vi "UI Enable & Disable.vi"(7 "Mode":T2(ring), 8 "error in (no error)":errorcluster, 11 "Ctl Refs In":T1) -> (0 "error out":errorcluster, 3 "Ctl Refs Out":T1)   [LabVIEW 2015]
doc: "VI that manages enabling & disabling certain portions of the UI under different sets of conditions."
uses:
  Type Defs/Control Refs.ctl
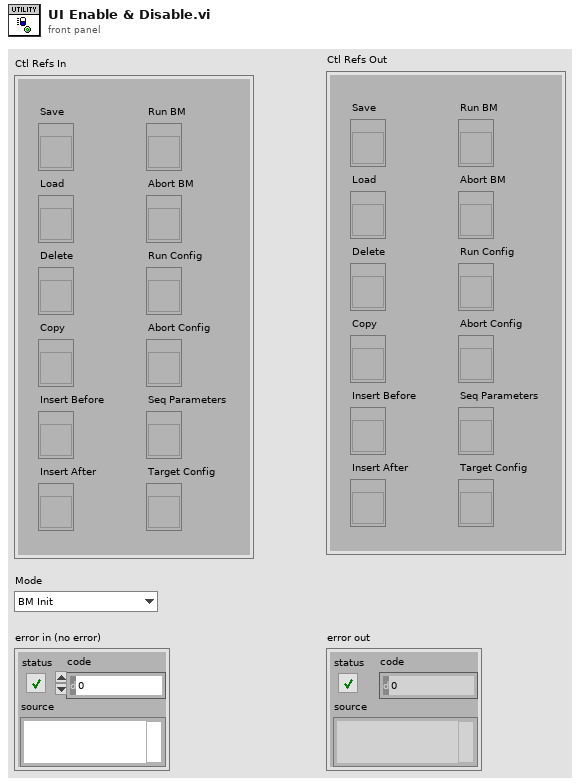
[diagram p1: front panel]
types:
  T1 = typedef "Control Refs.ctl" = cluster{"Save":refnum<vi>, "Load":refnum<vi>, "Delete":refnum<vi>, "Copy":refnum<vi>, "Insert Before":refnum<vi>, "Insert After":refnum<vi>, "Run BM":refnum<vi>, "Abort BM":refnum<vi>, "Run Config":refnum<vi>, "Abort Config":refnum<vi>, "Seq Parameters":refnum<vi>, "Target Config":refnum<vi>}
  T2 = enum16{"BM Init", "BM Run", "BM End", "Config Init", "Config Run", "Config End"}
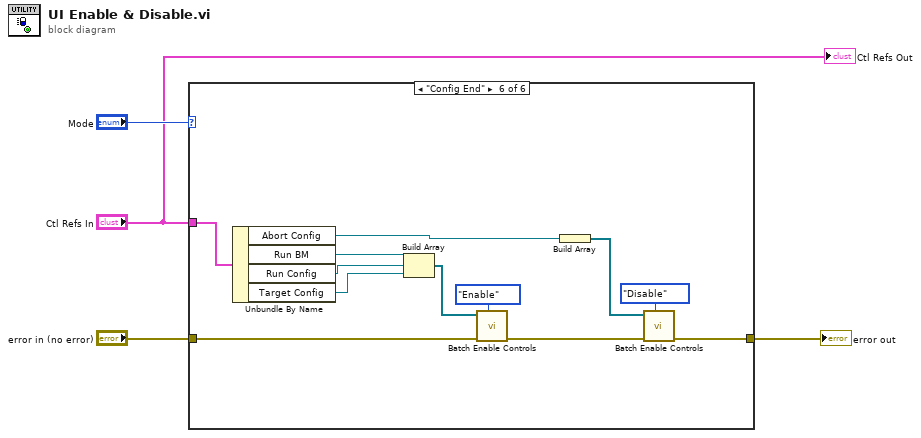
[diagram p0: block diagram]
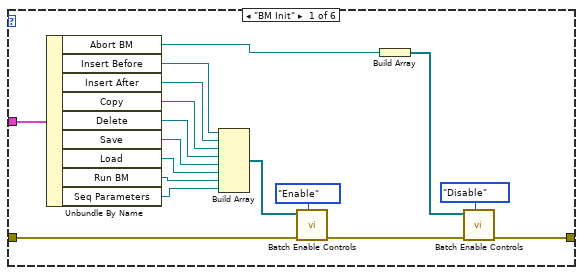
[diagram p2: hidden frame]
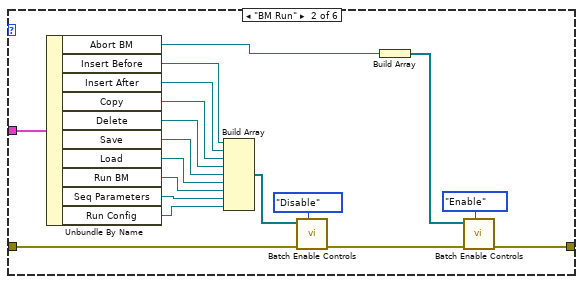
[diagram p3: hidden frame]
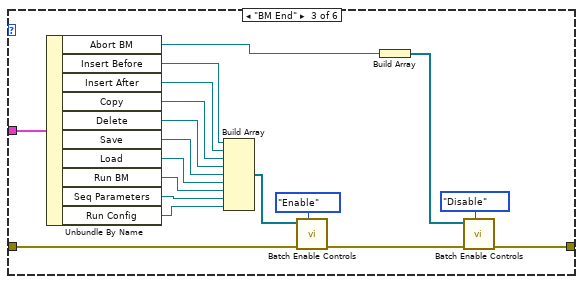
[diagram p4: hidden frame]
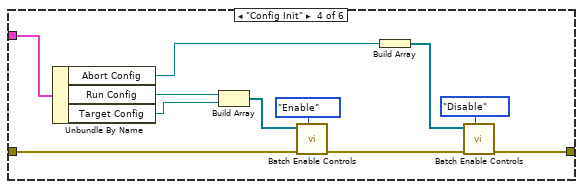
[diagram p5: hidden frame]
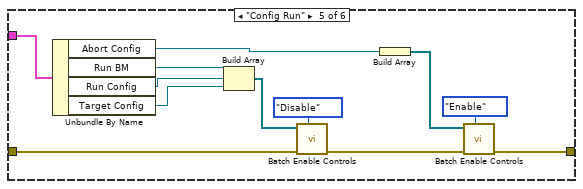
[diagram p6: hidden frame]
diagram:
  n1 = case shown="\"Config End\"" "Mode" {
    tunnel: "error in (no error)" -> [w21 w39 w57 w68 w80 w92]
    tunnel: "Ctl Refs In" -> [w19 w37 w55 w66 w78 w90]
    tunnel: [w5 w23 w41 w60 w74 w86] -> w2
    frame "BM Init" {
      n2 = Unbundle By Name(w19) -> ("Abort BM"=w8:refnum<vi>, "Insert Before"=w18:refnum<vi>, "Insert After"=w17:refnum<vi>, "Copy"=w16:refnum<vi>, "Delete"=w14:refnum<vi>, "Save"=w15:refnum<vi>, "Load"=w13:refnum<vi>, "Run BM"=w12:refnum<vi>, "Seq Parameters"=w11:refnum<vi>)
      n3 = Build Array(w18, w17, w16, w14, w15, w13, w12, w11) -> (w9:refnum<vi>[])
      n4 = call "Batch Enable Controls.vi"("Mode"=enum16{"Enable", "Disable"}."Enable", "error in (no error)"=w21, "Control Refs"=w9) -> ("error out"=w20:errorcluster)  [unwired: 8 in]
      n5 = Build Array(w8) -> (w6:refnum<vi>[])
      n6 = call "Batch Enable Controls.vi"("Mode"=enum16{"Enable", "Disable"}."Disable", "error in (no error)"=w20, "Control Refs"=w6) -> ("error out"=w5:errorcluster)  [unwired: 8 in]
    }
    frame "BM Run" {
      n7 = Unbundle By Name(w37) -> ("Abort BM"=w26:refnum<vi>, "Insert Before"=w36:refnum<vi>, "Insert After"=w35:refnum<vi>, "Copy"=w34:refnum<vi>, "Delete"=w32:refnum<vi>, "Save"=w33:refnum<vi>, "Load"=w31:refnum<vi>, "Run BM"=w30:refnum<vi>, "Seq Parameters"=w29:refnum<vi>, "Run Config"=w22:refnum<vi>)
      n8 = Build Array(w36, w35, w34, w32, w33, w31, w30, w29, w22) -> (w27:refnum<vi>[])
      n9 = call "Batch Enable Controls.vi"("Mode"=enum16{"Enable", "Disable"}."Disable", "error in (no error)"=w39, "Control Refs"=w27) -> ("error out"=w38:errorcluster)  [unwired: 8 in]
      n10 = Build Array(w26) -> (w24:refnum<vi>[])
      n11 = call "Batch Enable Controls.vi"("Mode"=enum16{"Enable", "Disable"}."Enable", "error in (no error)"=w38, "Control Refs"=w24) -> ("error out"=w23:errorcluster)  [unwired: 8 in]
    }
    frame "BM End" {
      n12 = Unbundle By Name(w55) -> ("Abort BM"=w44:refnum<vi>, "Insert Before"=w54:refnum<vi>, "Insert After"=w53:refnum<vi>, "Copy"=w52:refnum<vi>, "Delete"=w50:refnum<vi>, "Save"=w51:refnum<vi>, "Load"=w49:refnum<vi>, "Run BM"=w48:refnum<vi>, "Seq Parameters"=w47:refnum<vi>, "Run Config"=w40:refnum<vi>)
      n13 = Build Array(w54, w53, w52, w50, w51, w49, w48, w47, w40) -> (w45:refnum<vi>[])
      n14 = call "Batch Enable Controls.vi"("Mode"=enum16{"Enable", "Disable"}."Enable", "error in (no error)"=w57, "Control Refs"=w45) -> ("error out"=w56:errorcluster)  [unwired: 8 in]
      n15 = Build Array(w44) -> (w42:refnum<vi>[])
      n16 = call "Batch Enable Controls.vi"("Mode"=enum16{"Enable", "Disable"}."Disable", "error in (no error)"=w56, "Control Refs"=w42) -> ("error out"=w41:errorcluster)  [unwired: 8 in]
    }
    frame "Config Init" {
      n17 = Unbundle By Name(w66) -> ("Abort Config"=w59:refnum<vi>, "Run Config"=w65:refnum<vi>, "Target Config"=w58:refnum<vi>)
      n18 = Build Array(w65, w58) -> (w63:refnum<vi>[])
      n19 = call "Batch Enable Controls.vi"("Mode"=enum16{"Enable", "Disable"}."Enable", "error in (no error)"=w68, "Control Refs"=w63) -> ("error out"=w67:errorcluster)  [unwired: 8 in]
      n20 = Build Array(w59) -> (w61:refnum<vi>[])
      n21 = call "Batch Enable Controls.vi"("Mode"=enum16{"Enable", "Disable"}."Disable", "error in (no error)"=w67, "Control Refs"=w61) -> ("error out"=w60:errorcluster)  [unwired: 8 in]
    }
    frame "Config Run" {
      n22 = Unbundle By Name(w78) -> ("Abort Config"=w70:refnum<vi>, "Run BM"=w73:refnum<vi>, "Run Config"=w72:refnum<vi>, "Target Config"=w69:refnum<vi>)
      n23 = Build Array(w73, w72, w69) -> (w71:refnum<vi>[])
      n24 = call "Batch Enable Controls.vi"("Mode"=enum16{"Enable", "Disable"}."Disable", "error in (no error)"=w80, "Control Refs"=w71) -> ("error out"=w79:errorcluster)  [unwired: 8 in]
      n25 = Build Array(w70) -> (w75:refnum<vi>[])
      n26 = call "Batch Enable Controls.vi"("Mode"=enum16{"Enable", "Disable"}."Enable", "error in (no error)"=w79, "Control Refs"=w75) -> ("error out"=w74:errorcluster)  [unwired: 8 in]
    }
    frame "Config End" {
      n27 = Unbundle By Name(w90) -> ("Abort Config"=w82:refnum<vi>, "Run BM"=w85:refnum<vi>, "Run Config"=w84:refnum<vi>, "Target Config"=w81:refnum<vi>)
      n28 = Build Array(w85, w84, w81) -> (w83:refnum<vi>[])
      n29 = call "Batch Enable Controls.vi"("Mode"=enum16{"Enable", "Disable"}."Enable", "error in (no error)"=w92, "Control Refs"=w83) -> ("error out"=w91:errorcluster)  [unwired: 8 in]
      n30 = Build Array(w82) -> (w87:refnum<vi>[])
      n31 = call "Batch Enable Controls.vi"("Mode"=enum16{"Enable", "Disable"}."Disable", "error in (no error)"=w91, "Control Refs"=w87) -> ("error out"=w86:errorcluster)  [unwired: 8 in]
    }
  }
  "error out" <- w2
  "Ctl Refs Out" <- "Ctl Refs In"
